vi "Friedman1.vi"(8 "error in (no error)":errorcluster caption="entrée d'erreur (pas d'erreur)", 11 "make_friedman1":T2={"n_samples"=100, "n_features"=10, "noise"=0.0, "random_state"=-1, "Returns"="X"} {"n_features" min=5; "n_samples" min=1}) -> (0 "error out":errorcluster, 3 "Data":T1)   [LabVIEW 2020]
doc: "Generate the “Friedman #1” regression problem :\n\nThis dataset is described in Friedman [1] and Breiman [2].\n\nInputs X are independent features uniformly distributed on the interval [0, 1]. The output y is created according to the formula:\n\ny(X) = 10 * sin(pi * X[:, 0] * X[:, 1]) + 20 * (X[:, 2] - 0.5) ** 2 + 10 * X[:, 3] + 5 * X[:, 4] + noise * N(0, 1).\nOut of the n_features features, only 5 are actually used to compute y. The remaining features are independent of y.\n\nThe number of features has to be >= 5.\n\n\nParameters :\n\n- n_samples : int, optional (default=100)\nThe number of samples.\n\n- n_features : int, optional (default=10)\nThe number of features. Should be at least 5.\n\n- noise : float, optional (default=0.0)\nThe standard deviation of the gaussian noise applied to the output.\n\n- random_state : int, RandomState instance, default=None=-1\nDetermines random number generation for dataset noise. Pass an int for reproducible output across multiple function calls. See Glossary.\n\nReturns : \n\nX : array of shape [n_samples, n_features]\nThe input samples.\n\ny : array of shape [n_samples]\nThe output values"
uses:
  Friedman1.lvclass
panel:
  out "Friedman1.lvclass":refnum<class "Friedman1.lvclass">
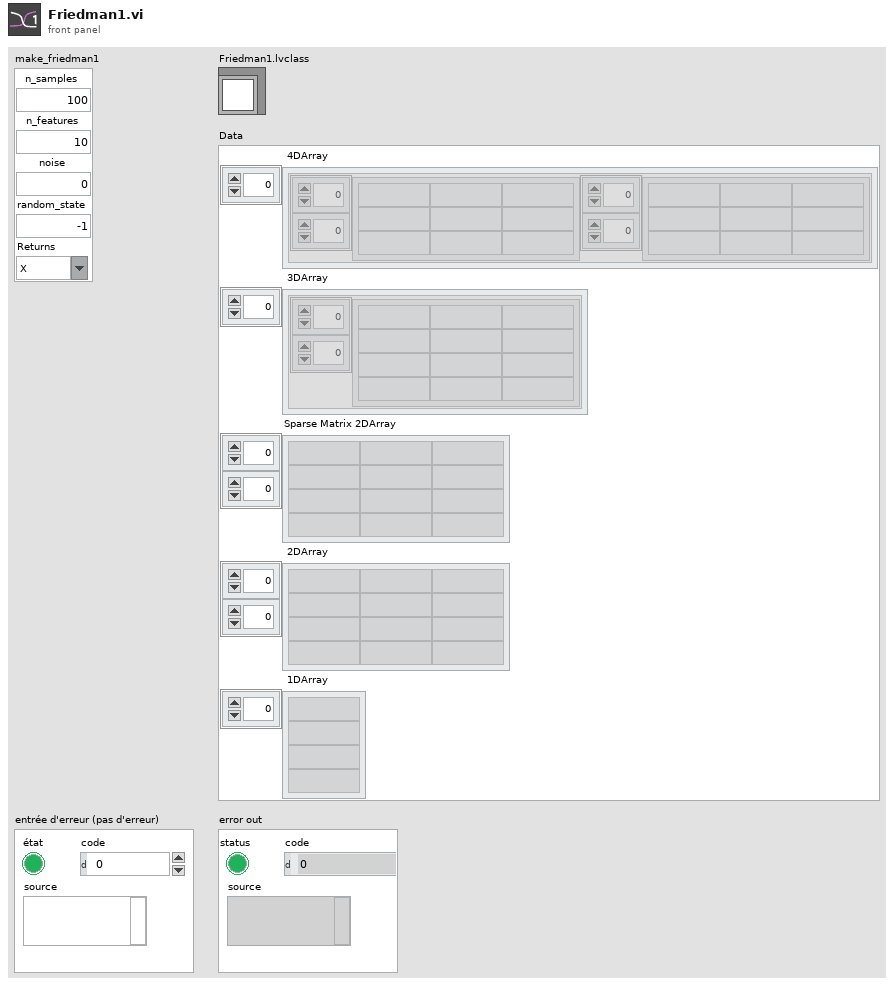
[diagram p1: front panel]
types:
  T1 = cluster{" 4DArray":cluster{"1":string[][], "2":string[][]}[], " 3DArray":cluster{"Tableau":string[][]}[], "Sparse Matrix 2DArray":string[][], " 2DArray":string[][], " 1DArray":string[]}
  T2 = cluster{"n_samples":u32, "n_features":u32, "noise":dbl, "random_state":i32, "Returns":string}
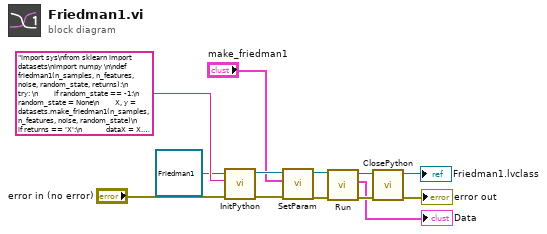
[diagram p0: block diagram]
diagram:
  n1 = call-dynamic "InitPython.vi"("error in (no error)"="error in (no error)", "Python Instruction"="import sys\nfrom sklearn import datasets\nimport numpy \n\ndef friedman1(n_samples, n_features, noise, random_state, returns):\n    try: \n        if random_state == -1:\n            random_state = None\n        X, y = datasets.make_friedman1(n_samples, n_features, noise, random_state)\n        if returns == 'X':\n            dataX = X.tolist()\n            return str(dataX)\n        else :\n            datay = y.tolist()\n            return str(datay)\n    except:\n        erreur = sys.exc_info()\n        typerr = u\"%s\" % (erreur[0])\n        typerr = typerr[typerr.find(\"'\")+1:typerr.rfind(\"'\")]\n        msgerr = u\"%s\" % (erreur[1])\n        message = str('/!\\\\ {0} : {1}'. format(typerr,msgerr))\n        return message", "Scikit-learn en entrée"=refnum<class "Friedman1.lvclass"> refnum ("Friedman1.lvclass")) -> ("error out"=w8:errorcluster, "Scikit-learn en sortie"=w7:refnum<class "Friedman1.lvclass">)  [unwired: 7 in]
  n2 = call-dynamic "SetParam.vi"("error in (no error)"=w8, "make_friedman1"="make_friedman1", "Friedman1.lvclass"=w7) -> ("error out"=w4:errorcluster, "Friedman1.lvclass"=w5:refnum<class "Friedman1.lvclass">)  [unwired: 7 in]
  n3 = call-dynamic "Run.vi"("error in (no error)"=w4, "Friedman1.lvclass"=w5) -> ("error out"=w10:errorcluster, "Data"=→"Data":T1, "Friedman1.lvclass"=w9:refnum<class "Friedman1.lvclass">)  [unwired: 7 in]
  n4 = call-dynamic "ClosePython.vi"("error in (no error)"=w10, "Scikit-learn en entrée"=w9) -> ("error out"=→"error out":errorcluster, "Scikit-learn en sortie"=→"Friedman1.lvclass":refnum<class "Friedman1.lvclass">)  [unwired: 8 in]
